vi "Perform Decimation Test (Enable Logging Then Open File).vi"(4 "Expected Group dts":dbl[](array[numeric]), 6 "Expected Y Array Sizes":i32[](array[numeric]), 7 "Decimation":dbl, 8 "error in":errorcluster, 9 "Embedded Data Logger Channel Group Name":string, 10 "Embedded Data Logger File Name":string, 11 "Embedded Data Logger Windows System Tests in":refnum<class "Embedded Data Logger Windows System Tests.lvclass">) -> (0 "error out":errorcluster, 3 "Embedded Data Logger Windows System Tests out":refnum<class "Embedded Data Logger Windows System Tests.lvclass">)   [LabVIEW 2027, in "Embedded Data Logger Windows System Tests.lvclass"]
uses:
  Embedded Data Logger Windows System Tests.lvclass
  b5d10dba-e1d4-49d3-a293-54a4a24a13a3.vi
  879fcf91-108b-492f-99e0-8bd5bbabdc7d.vi
  c4ab4416-d192-4b0f-97f0-08298a679134.vi
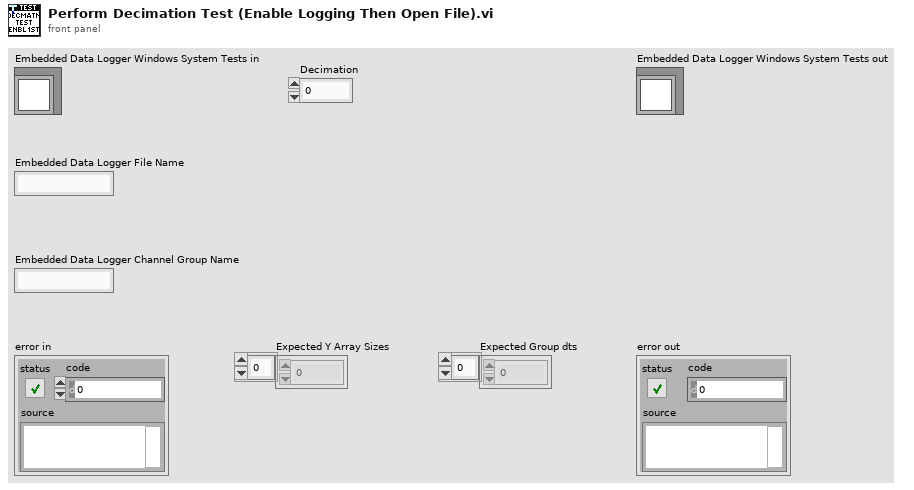
[diagram p1: front panel]
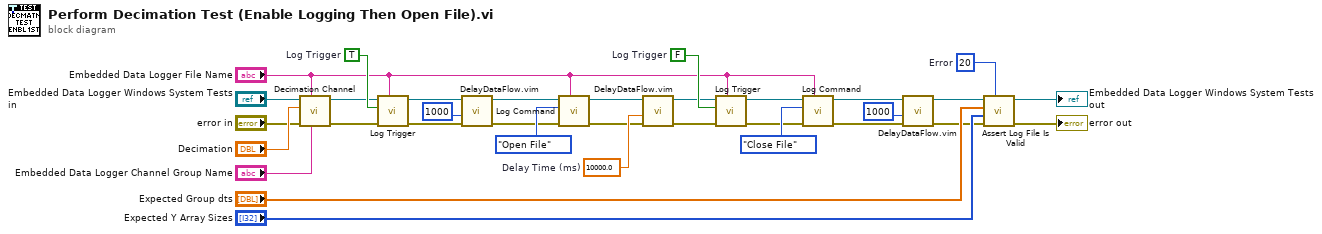
[diagram p0: block diagram]
diagram:
  w21 = 20  # Error
  w18 = FALSE  # Log Trigger
  w14 = 10000.0  # Delay Time (ms)
  w17 = TRUE  # Log Trigger
  n1 = call "Decimation Channel.vi"("Embedded Data Logger Channel Group Name"="Embedded Data Logger Channel Group Name", "Embedded Data Logger File Name"="Embedded Data Logger File Name", "error in"="error in", "Decimation"="Decimation", "Embedded Data Logger System Tests in"="Embedded Data Logger Windows System Tests in") -> ("error out"=w11:errorcluster, "Embedded Data Logger System Tests out"=w12:refnum<class "Embedded Data Logger Windows System Tests.lvclass">)  [unwired: 5 in]
  n2 = call "Log Trigger.vi"("Embedded Data Logger File Name"="Embedded Data Logger File Name", "error in"=w11, "Log Trigger"=w17, "Embedded Data Logger System Tests in"=w12) -> ("error out"=w5:errorcluster, "Embedded Data Logger System Tests out"=w10:refnum<class "Embedded Data Logger Windows System Tests.lvclass">)  [unwired: 6 in]
  n3 = call "DelayDataFlow.vim"("value in"=w5, "milliseconds to wait"=u32 1000) -> ("value out"=w4:errorcluster)  [unwired: 2 in, 1 out]
  n4 = call "Log Command.vi"("Embedded Data Logger File Name"="Embedded Data Logger File Name", "error in"=w4, "Log Command"=enum16{"Idle", "Open File", "Close File"}."Open File", "Embedded Data Logger System Tests in"=w10) -> ("error out"=w8:errorcluster, "Embedded Data Logger System Tests out"=w9:refnum<class "Embedded Data Logger Windows System Tests.lvclass">)  [unwired: 6 in]
  n5 = call "DelayDataFlow.vim"("value in"=w8, "milliseconds to wait"=w14) -> ("value out"=w13:errorcluster)  [unwired: 2 in, 1 out]
  n6 = call "Log Trigger.vi"("Embedded Data Logger File Name"="Embedded Data Logger File Name", "error in"=w13, "Log Trigger"=w18, "Embedded Data Logger System Tests in"=w9) -> ("error out"=w15:errorcluster, "Embedded Data Logger System Tests out"=w16:refnum<class "Embedded Data Logger Windows System Tests.lvclass">)  [unwired: 6 in]
  n7 = call "Log Command.vi"("Embedded Data Logger File Name"="Embedded Data Logger File Name", "error in"=w15, "Log Command"=enum16{"Idle", "Open File", "Close File"}."Close File", "Embedded Data Logger System Tests in"=w16) -> ("error out"=w2:errorcluster, "Embedded Data Logger System Tests out"=w19:refnum<class "Embedded Data Logger Windows System Tests.lvclass">)  [unwired: 6 in]
  n8 = call "DelayDataFlow.vim"("value in"=w2, "milliseconds to wait"=u32 1000) -> ("value out"=w1:errorcluster)  [unwired: 2 in, 1 out]
  n9 = call "Assert Log File Is Valid.vi"("Error"=w21, "error in"=w1, "Expected Y Array Sizes"="Expected Y Array Sizes", "Expected Group dts"="Expected Group dts", "Embedded Data Logger System Tests in"=w19) -> ("error out"=→"error out":errorcluster, "Embedded Data Logger System Tests out"=→"Embedded Data Logger Windows System Tests out":refnum<class "Embedded Data Logger Windows System Tests.lvclass">)  [unwired: 5 in]
